vi "testTTL_v3.vi"() -> ()   [LabVIEW 2015]
uses:
  <vilib>/DAQmx/read.llb/DAQmx Read (Counter U32 1Chan 1Samp).vi
  <vilib>/DAQmx/write.llb/DAQmx Write (Digital Bool 1Line 1Point).vi
  <vilib>/DAQmx/write.llb/DAQmx Write (Analog Wfm 1Chan NSamp).vi
  <vilib>/DAQmx/create/channels.llb/DAQmx Create Channel (CI-Count Edges).vi
  <vilib>/DAQmx/miscellaneous.llb/DAQmx Fill In Error Info.vi
  Windows/System32/kernel32.dll
  <resource>/objmgr/daqmx.rc
panel:
  out "sample count":u32
  out "OEP ms":dbl
  in  "Sample rate":dbl=30000.0
  in  "OEP sample clock in":tag="/Dev1/PFI1"
  in  "extra delay (ms)":dbl
  out "Curr delay (ms)":dbl(graph)
  out "max delay (ms)":dbl format="%#_10g"
  out "AO error out":errorcluster
  in  "Delay lock":bool
  out "wait time (ms)":dbl
  out "count 3":u64
  out "DO error out":errorcluster
  out "count 4":u64
  out "count 2":u64
  out "count 1":u64
  out "wait end to pulse gen end (ms)":dbl
  out "OEP to wait start (ms)":dbl caption="event rx to pulse gen start (ms)"
  out "time off (s)":dbl
  in  "Stop":bool
  out "level":sgl
  out "time on (s)":dbl
  out "New event":bool
  in  "event channel":u8=1 min=1 max=8
  out "ZMQ error out":errorcluster
  in  "error in":errorcluster
  in  "port":u16=5557
  # "Timing"
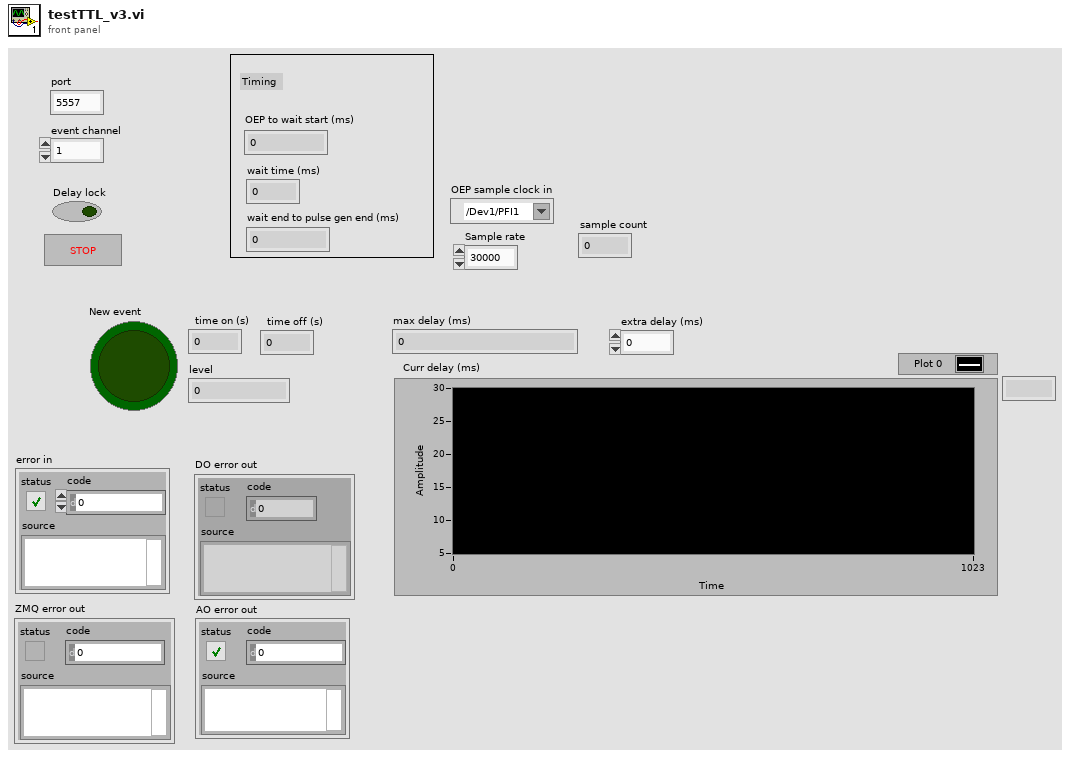
[diagram p1: front panel]
types:
  T1 = enum16{"big-endian, network order", "native, host order", "little-endian"}
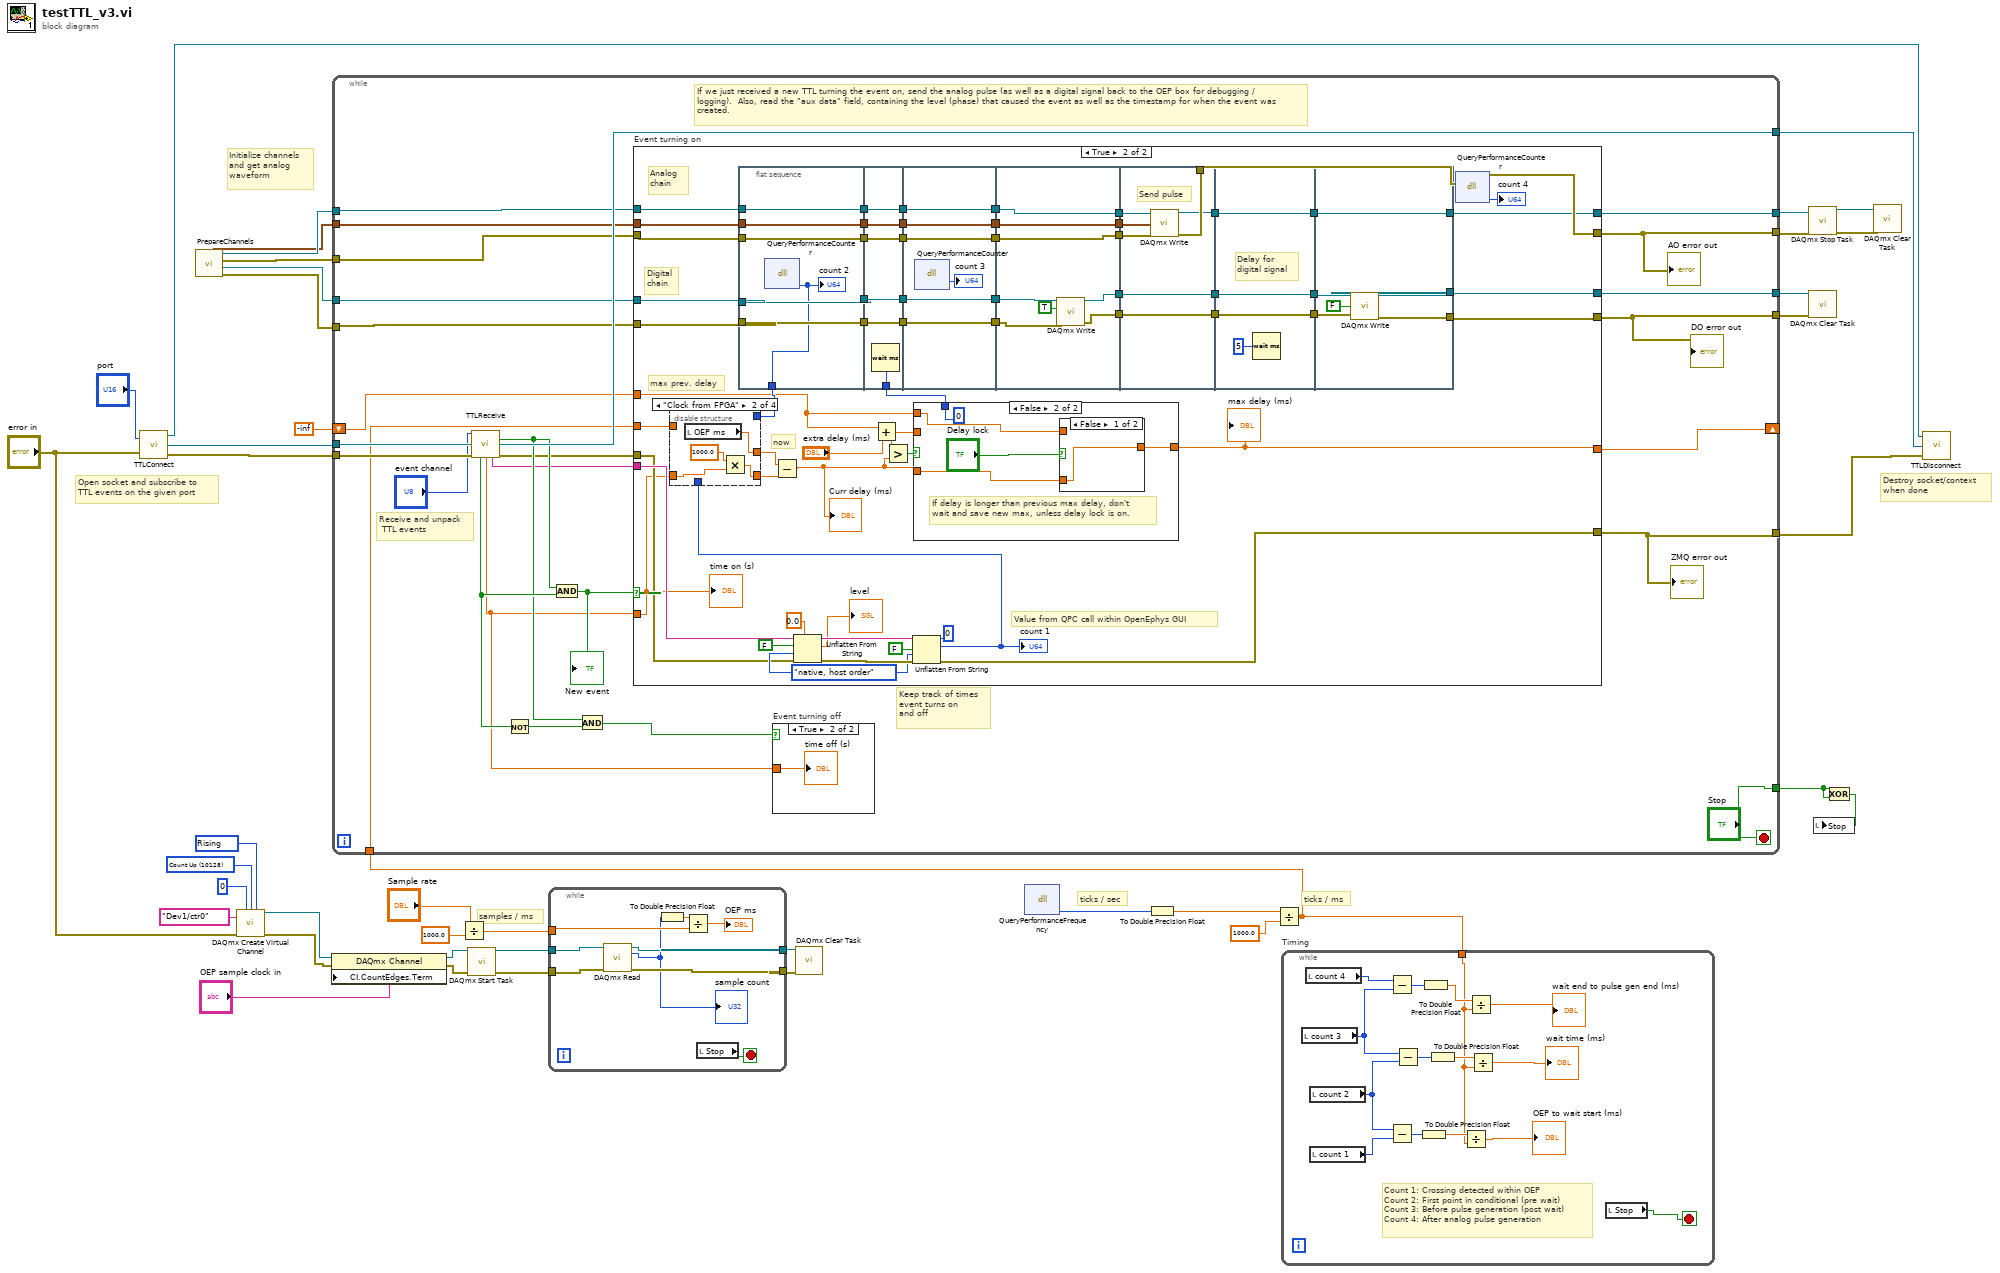
[diagram p0: block diagram]
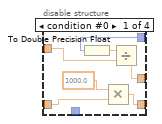
[diagram p3: hidden frame]
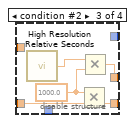
[diagram p4: hidden frame]
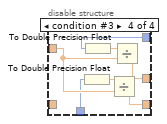
[diagram p5: hidden frame]
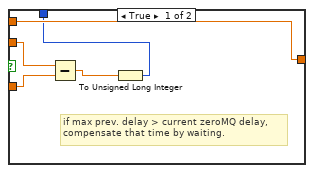
[diagram p6: hidden frame]
diagram:
  w12 = 10280 items=["Rising"=10280, "Falling"=10171] ("edge")
  w13 = 10128 items=["Count Up"=10128, "Count Down"=10124, "Externally Controlled"=10326] ("count direction")
  # "samples / ms"
  # "Initialize channels\nand get analog\nwaveform"
  # "ticks / ms"
  # "ticks / sec"
  # "Open socket and subscribe to\nTTL events on the given port"
  # "Destroy socket/context\nwhen done"
  n1 = call "TTLConnect.vi"("port"="port", "error in"="error in") -> ("context out"=w40:refnum<class "zmq_context.lvclass">, "socket out"=w24:refnum<class "zmq_socket.lvclass">, "error out"=w25:errorcluster)
  n2 = call "PrepareChannels.vi"() -> ("DO error out"=w36:errorcluster, "DO task out"=w37:refnum<k21>, "AO error out"=w35:errorcluster, "AO task out"=w38:refnum<k21>, "Waveform Graph"=w30:waveform(dbl))  [unwired: 7 in]
  n3 = call-poly <vilib>:"DAQmx Create Virtual Channel.vi"("initial count"=u32 0, "count direction"=w13, "edge"=w12, "counter"=tag "Dev1/ctr0", "error in"="error in") -> ("task out"=w17:refnum<k21>, "error out"=w16:errorcluster)  [unwired: 9 in]
  n4 = property class="DAQmx Channel"(reference=w17, error in=w16, "CI.CountEdges.Term"="OEP sample clock in") -> (reference out=w11:refnum<k21>, error out=w10:errorcluster)
  n5 = Divide(x="Sample rate", y=1000.0) -> (x/y=w1:dbl)
  n6 = call <vilib>:"DAQmx Start Task.vi"("task/channels in"=w11, "error in"=w10) -> ("task out"=w8:refnum<k21>, "error out"=w7:errorcluster)  [unwired: 12 in]
  n7 = while {
    tunnel: w8 -> [w49]
    tunnel: w7 -> [w48]
    tunnel: [w47] -> w6
    tunnel: [w46] -> w5
    tunnel: w1 -> [w45]
    stop <- w50 stop-if-true
    n8 = call-poly <vilib>:"DAQmx Read.vi"("task/channels in"=w49, "error in"=w48) -> ("task out"=w46:refnum<k21>, "data"=w43:u32, "error out"=w47:errorcluster)  [unwired: 11 in]
    "sample count" <- w43
    n9 = To Double Precision Float(number=w43) -> (double precision float=w44:dbl)
    n10 = Divide(x=w44, y=w45) -> (x/y=→"OEP ms":dbl)
    n11 = local read "Stop"() -> (w50:bool)
  }
  n12 = call <vilib>:"DAQmx Clear Task.vi"("task in"=w5, "error in"=w6) -> ()  [unwired: 13 in, 1 out]
  n13 = dll-call lib="C:/Windows/System32/kernel32.dll" fn="QueryPerformanceFrequency"() -> ("lpFrequency"=w22:u64)  [unwired: 5 in, 2 out]
  n14 = To Double Precision Float(number=w22) -> (double precision float=w19:dbl)
  n15 = Divide(x=w19, y=1000.0) -> (x/y=w18:dbl)
  n16 = while {
    tunnel: w25 -> [w76]
    tunnel: [w52] -> w23
    tunnel: [w75] -> w39
    tunnel: w24 -> [w74]
    tunnel: w38 -> [w71]
    tunnel: w37 -> [w69]
    tunnel: w36 -> [w68]
    tunnel: w35 -> [w70]
    tunnel: [w57] -> w29
    tunnel: [w56] -> w28
    tunnel: [w60] -> w34
    tunnel: [w53] -> w33
    tunnel: ["Stop"] -> w32
    tunnel: w30 -> [w58]
    shift-right: [w54] -> _
    shift-left: -inf -> [w55]
    tunnel: w18 -> [w51]
    stop <- "Stop" stop-if-true
    # "Receive and unpack\n TTL events"
    # "If we just received a new TTL turning the event on, send the analog pulse (as well as a digital signal back to the OEP box for debugging / logging).  Also, read the \"aux data\" field, containing the level (phase) that caused the event as well as the timestamp for when the event was created."
    # "Keep track of times\nevent turns on\nand off"
    n17 = call "TTLReceive.vi"("channel"="event channel", "socket in"=w74, "error in"=w76) -> ("new TTL"=w65:bool, "socket out"=w75:refnum<class "zmq_socket.lvclass">, "event on"=w66:bool, "timestamp (s)"=w63:dbl, "aux data"=w62:string, "error out"=w61:errorcluster)  [unwired: 6 in, 1 out]
    n18 = Not(x=w66) -> (.not. x?=w67:bool)
    n19 = And(x=w65, y=w66) -> (x .and. y?=w72:bool)
    "New event" <- w72
    n20 = And(x=w65, y=w67) -> (x .and. y?=w64:bool)
    n21 = case "Event turning on" shown="True" w72 {
      tunnel: w71 -> [w82 w120]
      tunnel: w70 -> [w81 w104]
      tunnel: [w82 w118] -> w57
      tunnel: [w81 w124] -> w56
      tunnel: w69 -> [w79 w142]
      tunnel: w68 -> [w78 w125]
      tunnel: [w79 w143] -> w60
      tunnel: [w78 w129] -> w53
      tunnel: w63 -> [_ w92]
      tunnel: w62 -> [_ w134]
      tunnel: w61 -> [w80 w132]
      tunnel: [w80 w133] -> w52
      tunnel: w58 -> [_ w121]
      tunnel: w55 -> [w77 w86]
      tunnel: [w77 w127] -> w54
      tunnel: w51 -> [_ w90]
      frame False {
      }
      frame True {
        w136 = T1."native, host order" ("byte order (0:big-endian, network order)")
        # "now"
        # "Digital\nchain"
        # "Analog \nchain"
        # "Value from QPC call within OpenEphys GUI"
        # "max prev. delay"
        n22 = flat-sequence {
          tunnel: w120 -> [w180]
          tunnel: w121 -> [w181]
          tunnel: w104 -> [w182]
          tunnel: w125 -> [w183]
          tunnel: w142 -> [w184]
          tunnel: [w184] -> w109
          tunnel: [w183] -> w108
          tunnel: [w182] -> w107
          tunnel: [w181] -> w106
          tunnel: [w180] -> w105
          tunnel: [w179] -> w87
          tunnel: [w188] -> w103
          tunnel: [w190] -> w101
          tunnel: w126 -> [w189]
          tunnel: [w187] -> w99
          tunnel: [w186] -> w97
          tunnel: [w185] -> w95
          tunnel: w109 -> [w190]
          tunnel: w108 -> [w188]
          tunnel: w107 -> [w187]
          tunnel: w106 -> [w186]
          tunnel: w105 -> [w185]
          tunnel: w103 -> [w196]
          tunnel: [w196] -> w102
          tunnel: w101 -> [w195]
          tunnel: [w195] -> w100
          tunnel: w99 -> [w194]
          tunnel: [w194] -> w98
          tunnel: w97 -> [w193]
          tunnel: [w193] -> w96
          tunnel: w95 -> [w192]
          tunnel: [w192] -> w94
          tunnel: [w202] -> w117
          tunnel: [w201] -> w115
          tunnel: w102 -> [w197]
          tunnel: w100 -> [w203]
          tunnel: w98 -> [w200]
          tunnel: w96 -> [w198]
          tunnel: w94 -> [w199]
          tunnel: [w200] -> w112
          tunnel: [w199] -> w111
          tunnel: [w198] -> w110
          tunnel: w117 -> [w211]
          tunnel: [w211] -> w116
          tunnel: w115 -> [w210]
          tunnel: [w210] -> w114
          tunnel: [w205] -> w113
          tunnel: w112 -> [w208]
          tunnel: w111 -> [w206]
          tunnel: w110 -> [w209]
          tunnel: [w207] -> w93
          tunnel: [w215] -> w131
          tunnel: w116 -> [w215]
          tunnel: [w214] -> w130
          tunnel: w114 -> [w214]
          tunnel: w113 -> [w212]
          tunnel: [w212] -> w119
          tunnel: [w219] -> w143
          tunnel: w131 -> [w220]
          tunnel: w130 -> [w218]
          tunnel: [w217] -> w129
          tunnel: w119 -> [w216]
          tunnel: [w216] -> w118
          frame #0 {
            n23 = dll-call lib="C:/Windows/System32/kernel32.dll" fn="QueryPerformanceCounter" label="QPC"() -> ("lpPerformanceCount"=w179:u64)  [unwired: 5 in, 2 out]
            "count 2" <- w179
          }
          frame #1 {
            n24 = Wait (ms)(milliseconds to wait=w189) -> ()  [unwired: 1 out]
          }
          frame #2 {
            n25 = dll-call lib="C:/Windows/System32/kernel32.dll" fn="QueryPerformanceCounter" label="QPC"() -> ("lpPerformanceCount"=→"count 3":u64)  [unwired: 5 in, 2 out]
          }
          frame #3 {
            n26 = call-poly <vilib>:"DAQmx Write.vi"("task/channels in"=w203, "data"=TRUE, "error in"=w197) -> ("task out"=w202:refnum<k21>, "error out"=w201:errorcluster)  [unwired: 10 in, 1 out]
          }
          frame #4 {
            # "Send pulse"
            n27 = call-poly <vilib>:"DAQmx Write.vi"("task/channels in"=w206, "data"=w209, "error in"=w208) -> ("task out"=w205:refnum<k21>, "error out"=w207:errorcluster)  [unwired: 10 in, 1 out]
          }
          frame #5 {
            # "Delay for \ndigital signal"
            n28 = Wait (ms)(milliseconds to wait=u32 5) -> ()  [unwired: 1 out]
          }
          frame #6 {
            n29 = call-poly <vilib>:"DAQmx Write.vi"("task/channels in"=w220, "data"=FALSE, "error in"=w218) -> ("task out"=w219:refnum<k21>, "error out"=w217:errorcluster)  [unwired: 10 in, 1 out]
          }
        }
        n30 = Unflatten From String(type=sgl 0.0, binary string=w134, data includes array or string size? (T)=FALSE, byte order (0:big-endian, network order)=w136, error in (no error)=w132) -> (rest of the binary string=w138:string, value=→"level":sgl, error out=w139:errorcluster)
        n31 = Add(x=w86, y="extra delay (ms)") -> (x+y=w84:dbl)
        n32 = Unflatten From String(type=u64 0, binary string=w138, data includes array or string size? (T)=FALSE, byte order (0:big-endian, network order)=w136, error in (no error)=w139) -> (value=w91:u64, error out=w133:errorcluster)  [unwired: 1 out]
        "count 1" <- w91
        n33 = disable-structure shown="\"Clock from FPGA\"" {
          disable-tunnel: [w147 w151 w159 w166] -> w89
          disable-tunnel: w92 -> [w144 w153 w156 _]
          disable-tunnel: [w146 w152 w158 w165] -> w88
          disable-tunnel: w91 -> [_ _ _ w160]
          disable-tunnel: w90 -> [w148 _ _ w164]
          disable-tunnel: w87 -> [w149 _ _ w161]
          frame condition #0 {
            n34 = To Double Precision Float(number=w149) -> (double precision float=w150:dbl)
            n35 = Multiply(x=1000.0, y=w144) -> (x*y=w146:dbl)
            n36 = Divide(x=w150, y=w148) -> (x/y=w147:dbl)
          }
          frame condition #1 (active) {
            n37 = local read "OEP ms"() -> (w151:dbl)
            n38 = Multiply(x=1000.0, y=w153) -> (x*y=w152:dbl)
          }
          frame condition #2 {
            w155 = 1000.0 ("x")
            n39 = call <vilib>:"High Resolution Relative Seconds.vi"() -> ("relative seconds"=w157:dbl)
            n40 = Multiply(x=w155, y=w156) -> (x*y=w158:dbl)
            n41 = Multiply(x=w157, y=w155) -> (x*y=w159:dbl)
          }
          frame condition #3 {
            n42 = To Double Precision Float(number=w160) -> (double precision float=w163:dbl)
            n43 = To Double Precision Float(number=w161) -> (double precision float=w162:dbl)
            n44 = Divide(x=w163, y=w164) -> (x/y=w165:dbl)
            n45 = Divide(x=w162, y=w164) -> (x/y=w166:dbl)
          }
        }
        n46 = Subtract(x=w89, y=w88) -> (x-y=w83:dbl)
        "Curr delay (ms)" <- w83
        n47 = Greater?(x=w84, y=w83) -> (0:w128:bool)
        n48 = case shown="False" w128 {
          tunnel: w83 -> [w170 w173]
          tunnel: w86 -> [w171 w174]
          tunnel: [w171 w172] -> w127
          tunnel: [w169 u32 0] -> w126
          tunnel: w84 -> [w167 _]
          frame True {
            # "if max prev. delay > current zeroMQ delay,\ncompensate that time by waiting."
            n49 = Subtract(x=w167, y=w170) -> (x-y=w168:dbl)
            n50 = To Unsigned Long Integer(number=w168) -> (unsigned 32bit integer=w169:u32)
          }
          frame False, Default {
            # "If delay is longer than previous max delay, don't\nwait and save new max, unless delay lock is on."
            n51 = case shown="False" "Delay lock" {
              tunnel: w174 -> [_ w178]
              tunnel: w173 -> [w177 _]
              tunnel: [w177 w178] -> w172
              frame False {
              }
              frame True {
              }
            }
          }
        }
        "max delay (ms)" <- w127
        n52 = dll-call lib="C:/Windows/System32/kernel32.dll" fn="QueryPerformanceCounter" label="QPC"(error in=w93) -> (error out=w124:errorcluster, "lpPerformanceCount"=→"count 4":u64)  [unwired: 4 in, 1 out]
        "time on (s)" <- w92
      }
    }
    "DO error out" <- w53
    "AO error out" <- w56
    "ZMQ error out" <- w52
    n53 = case "Event turning off" shown="True" w64 {
      tunnel: w63 -> [_ w222]
      frame False {
      }
      frame True {
        "time off (s)" <- w222
      }
    }
  }
  n54 = while "Timing" {
    tunnel: w18 -> [w224]
    stop <- w231 stop-if-true
    # "Count 1: Crossing detected within OEP\nCount 2: First point in conditional (pre wait)\nCount 3: Before pulse generation (post wait)\nCount 4: After analog pulse generation"
    n55 = local read "count 3"() -> (w228:u64)
    n56 = local read "count 4"() -> (w237:u64)
    n57 = local read "count 2"() -> (w227:u64)
    n58 = local read "count 1"() -> (w232:u64)
    n59 = Subtract(x=w237, y=w228) -> (x-y=w236:u64)
    n60 = Subtract(x=w227, y=w232) -> (x-y=w235:u64)
    n61 = Subtract(x=w228, y=w227) -> (x-y=w226:u64)
    n62 = To Double Precision Float(number=w235) -> (double precision float=w233:dbl)
    n63 = To Double Precision Float(number=w236) -> (double precision float=w234:dbl)
    n64 = To Double Precision Float(number=w226) -> (double precision float=w225:dbl)
    n65 = Divide(x=w233, y=w224) -> (x/y=→"OEP to wait start (ms)":dbl)
    n66 = Divide(x=w234, y=w224) -> (x/y=→"wait end to pulse gen end (ms)":dbl)
    n67 = Divide(x=w225, y=w224) -> (x/y=→"wait time (ms)":dbl)
    n68 = local read "Stop"() -> (w231:bool)
  }
  n69 = call <vilib>:"DAQmx Stop Task.vi"("task/channels in"=w29, "error in"=w28) -> ("task out"=w27:refnum<k21>, "error out"=w26:errorcluster)  [unwired: 12 in]
  n70 = call <vilib>:"DAQmx Clear Task.vi"("task in"=w34, "error in"=w33) -> ()  [unwired: 13 in, 1 out]
  n71 = Exclusive Or(1:w32, 2:w32) -> (0:w31:bool)
  n72 = local write "Stop"(w31) -> ()
  n73 = call <vilib>:"DAQmx Clear Task.vi"("task in"=w27, "error in"=w26) -> ()  [unwired: 13 in, 1 out]
  n74 = call "TTLDisconnect.vi"("error in"=w23, "socket in"=w39, "context in"=w40) -> ()  [unwired: 1 in, 1 out]
